vi "TI_MSP430-Gamepad-test.vi"() -> ()   [LabVIEW 2019]
uses:
  <vilib>/Rock Robotics/WPI/Joystick/WPI_JoystickDeviceEnum.ctl
panel:
  in  "output 1":bool
  in  "output 2":bool
  out "outputs":bool[](array[boolean])
  out "wrt err":errorcluster
  out "read err":errorcluster
  in  "output 5":bool
  out "POVs":i16[](array[numeric])
  out "Buttons":bool[](array[boolean])
  out "Axes":dbl[](array[numeric])
  in  "JoystickDevice":T1
  # "Wiring   :\n    Inputs   --- 3.3V  ---- Button ----- Input terminal\n    outputs  --- output terminal  ---- 1k resistor --- LED ----- Gnd"
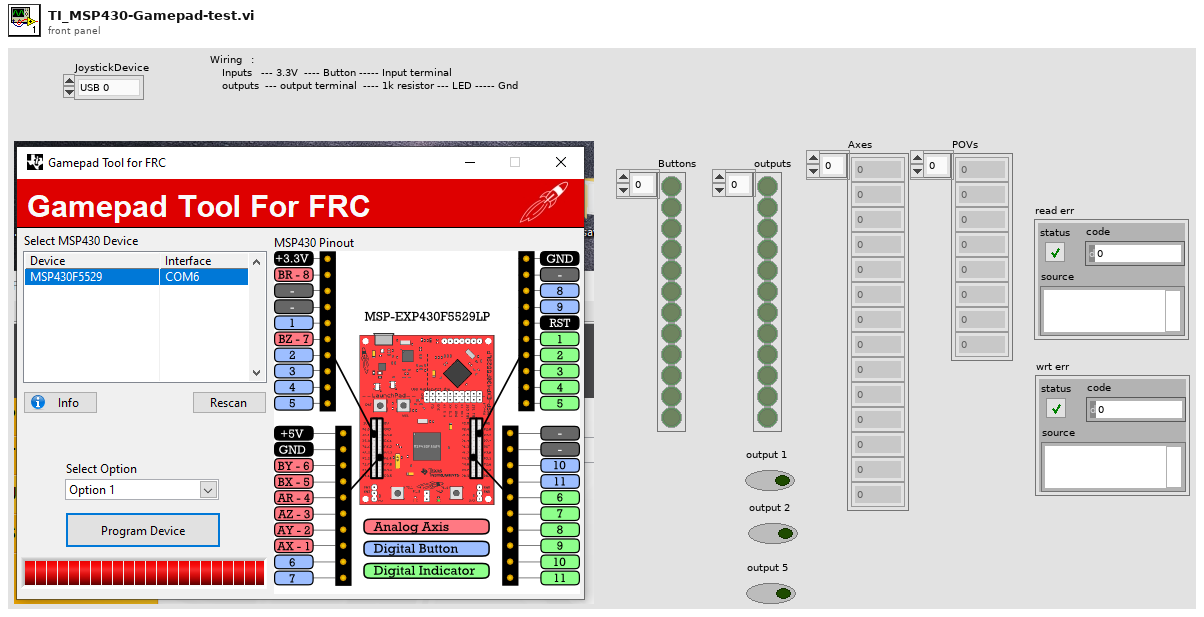
[diagram p1: front panel]
types:
  T1 = typedef "WPI_JoystickDeviceEnum.ctl" = enum16{"USB 0", "USB 1", "USB 2", "USB 3", "USB 4", "USB 5"}
  T2 = typedef "WPI_JoystickDevRef.ctl" = cluster{"Device":T1}
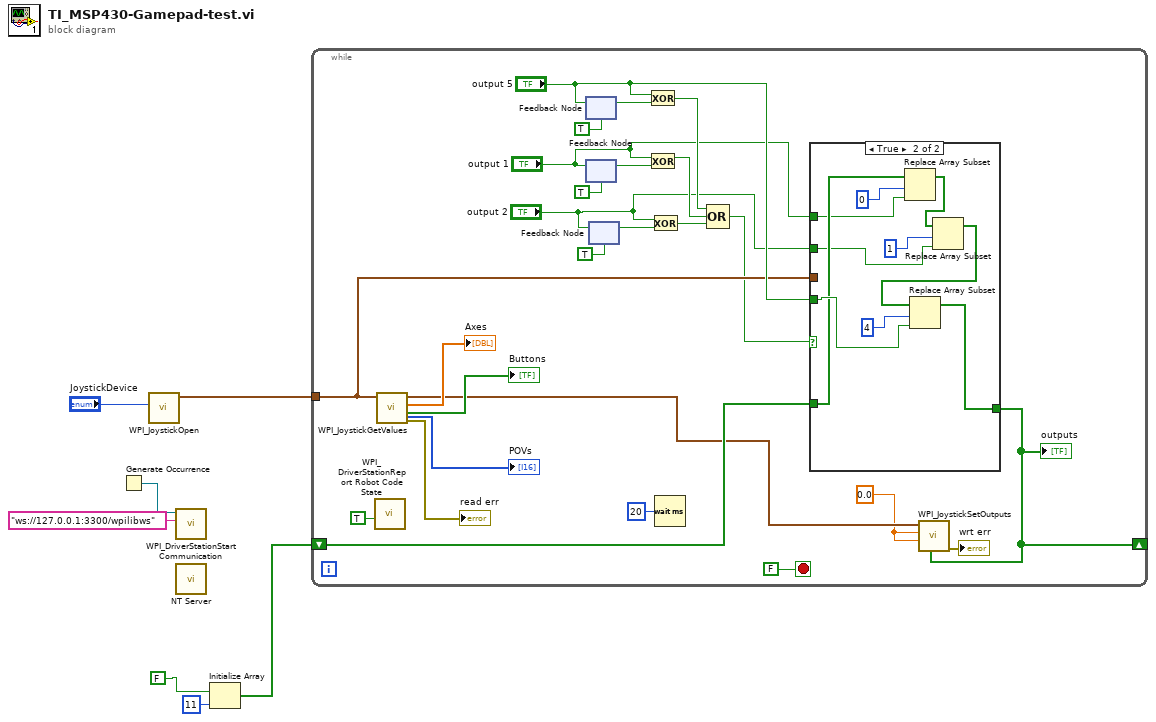
[diagram p0: block diagram]
diagram:
  n1 = Generate Occurrence() -> (w5:refnum<k4>)
  n2 = call <vilib>:"WPI_JoystickOpen.vi"("JoystickDevice"="JoystickDevice") -> ("JoystickDevRef"=w6:T2)  [unwired: 10 in]
  n3 = call <vilib>:"WPI_DriverStationStart Communication.vi"("Simulation URL"="ws://127.0.0.1:3300/wpilibws", "occurrence"=w5) -> ()  [unwired: 10 in]
  n4 = call <vilib>:"NT Server.vi"() -> ()  [unwired: 11 in, 1 out]
  n5 = Initialize Array(FALSE, 11 ("dimension size")) -> (w1:bool[])
  n6 = while {
    tunnel: w6 -> [w24]
    shift-right: [w8] -> _
    shift-left: w1 -> [w23]
    stop <- FALSE stop-if-true
    w9 = sgl 0.0 ("Left Rumble")
    n7 = call <vilib>:"WPI_DriverStationReport Robot Code State.vi"("TeleOp"=TRUE) -> ()  [unwired: 10 in, 1 out]
    n8 = call <vilib>:"WPI_JoystickGetValues.vi"("JoystickDevRef"=w24) -> ("error out"=→"read err":errorcluster, "Buttons"=→"Buttons":bool[], "Axes"=→"Axes":dbl[], "JoystickDevRef"=w10:T2, "POVs"=→"POVs":i16[])  [unwired: 6 in]
    n9 = feedback-in #1("output 5") -> ()
    n10 = feedback #1(TRUE ("Boolean")) -> (w27:bool)
    n11 = feedback #2(TRUE ("Boolean")) -> (w21:bool)
    n12 = feedback-in #2("output 1") -> ()
    n13 = feedback #3(TRUE ("Boolean")) -> (w19:bool)
    n14 = feedback-in #3("output 2") -> ()
    n15 = Exclusive Or(1:w27, 2:"output 5") -> (0:w15:bool)
    n16 = Exclusive Or(1:w21, 2:"output 1") -> (0:w16:bool)
    n17 = Exclusive Or(1:w19, 2:"output 2") -> (0:w17:bool)
    n18 = Wait (ms)(milliseconds to wait=u32 20) -> ()  [unwired: 1 out]
    n19 = Compound Arithmetic op=OR(w15, w16, w17) -> (w14:bool)
    n20 = case shown="True" w14 {
      tunnel: "output 5" -> [_ w43]
      tunnel: w24 -> [_ _]
      tunnel: w23 -> [w34 w39]
      tunnel: [w34 w42] -> w8
      tunnel: "output 1" -> [_ w36]
      tunnel: "output 2" -> [_ w35]
      frame False {
      }
      frame True {
        n21 = Replace Array Subset(array=w39, new element=w36, index=0) -> (w38:bool[])
        n22 = Replace Array Subset(array=w38, new element=w35, index=1) -> (w37:bool[])
        n23 = Replace Array Subset(array=w37, new element=w43, index=4) -> (w42:bool[])
      }
    }
    "outputs" <- w8
    n24 = call <vilib>:"WPI_JoystickSetOutputs.vi"("Outputs"=w8, "Right Rumble"=w9, "Left Rumble"=w9, "JoystickDevRef"=w10) -> ("error out"=→"wrt err":errorcluster)  [unwired: 6 in, 1 out]
  }
